vi "niDTS BT LE Rx Test  Initialize.vi"(0 "Dut Reference":T3, 5 "SystemTechnologyCatalog":refnum<class "niDTS SystemTechnologyCatalog.lvclass">, 7 "SystemDut":refnum<class "niDTS SystemDut.lvclass">, 9 "Logger Reference":T1, 11 "error in (no error)":errorcluster) -> (4 "RX Test Handle Out":T2, 6 "AllowAsync":bool=TRUE, 15 "error out":errorcluster)   [LabVIEW 2014, in "niDTS BT.lvlib"]
uses:
  niDTS BT.lvlib
  Framework/Dut/Includes/niDTS Dut INC Handle.ctl
  Framework/Dut/Objects/BASE_class/niDTS Dut.lvclass
  BDR Tx Test/Includes/niDTS BT Rx Test INC Handle.ctl
  Rx Test/Objects/BASE_class/niDTS BT Rx Test.lvclass
  TestStand/Station/Objects/SystemTechnologyCatalog/niDTS SystemTechnologyCatalog.lvclass
  TestStand/Station/Objects/SystemDut/niDTS SystemDut.lvclass
  Framework/Logger/Includes/niDTS Logger INC Handle.ctl
  Framework/Logger/Objects/BASE_class/niDTS Logger.lvclass
  Includes/niDTS BT INC Standard.ctl
  TestStand/niDTS TestStand.lvlib
  Framework/niDTS Framework.lvlib
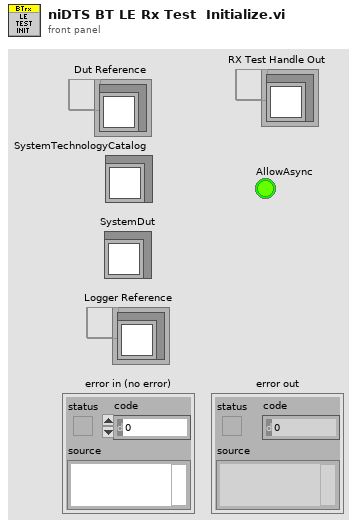
[diagram p1: front panel]
types:
  T1 = typedef "niDTS Framework.lvlib/niDTS Logger INC Handle.ctl" = refnum<data-value>
  T2 = typedef "niDTS BT.lvlib/niDTS BT Rx Test INC Handle.ctl" = refnum<data-value>
  T3 = typedef "niDTS Framework.lvlib/niDTS Dut INC Handle.ctl" = refnum<data-value>
  T4 = typedef "niDTS BT.lvlib/niDTS BT INC Standard.ctl" = enum16{"BDR", "EDR", "LE-TP"}
  T5 = typedef "niDTS TestStand.lvlib/niDTS TestStep INC Handle.ctl" = refnum<data-value>
  T6 = typedef "niDTS BT.lvlib/niDTS BT Rx Test INC Parameters.ctl" = cluster{"Channel":i32, "Dut Tx Power":dbl, "External Attenuation (dB)":dbl[], "Data Rate":enum16{"1", "2", "3"}, "Packet type":T7, "Payload Data":T8, "Carrier Mode":T9, "Number of Packets":i32, "Report Period (ms)":dbl, "BD ADDRESS":i64, "Dirty Tx":bool, "Corrupt Alternate CRC":bool, "Packet Header":T10, "Payload Header":T11, "Trigger":T12}
  T7 = typedef "niDTS BT.lvlib/niDTS BT INC Packet Type.ctl" = enum16{"NULL", "POLL", "FHS", "DM1", "DH1", "HV1", "HV2", "HV3", "EV3", "DV", "AUX1", "DM3", "DH3", "EV4", "EV5", "DM5", "DH5", "LE-TP"}
  T8 = typedef "niDTS BT.lvlib/niDTS BT Tx Test INC BD Payload Data.ctl" = enum16{"0", "1", "01", "00001111", "PN9", "AUTO"}
  T9 = typedef "niDTS BT.lvlib/niDTS BT Rx Test INC Carrier Mode.ctl" = enum16{"Burst", "Continuous"}
  T10 = typedef "niDTS BT.lvlib/niDTS BT Rx Test INC Packet Header.ctl" = cluster{"LT Address":i8, "Flow":i8, "ARQN":enum16{"NAK", "ACK"}, "Sequence Bit":i8}
  T11 = typedef "niDTS BT.lvlib/niDTS BT Rx Test INC Payload Header.ctl" = cluster{"LCh":i32, "HeaderFlowControlBit":bool, "Length (-1 AutoSet Max)":i32}
  T12 = typedef "niDTS BT.lvlib/niDTS BT DUT INC SG Trigger.ctl" = cluster{"TriggerEdge":enum16{"RISing", "FALLing"}, "TriggerSource":enum16{"IMMediate", "PFI 0", "PFI 1", "RTSI 0", "RTSI 1", "RTSI 2", "RTSI 3", "RTSI 4", "RTSI 5", "RTSI 6", "RTSI 7", "PXI STAR", "Software"}, "TriggerDelay (sec)":dbl, "TriggerTimeout (sec)":dbl}
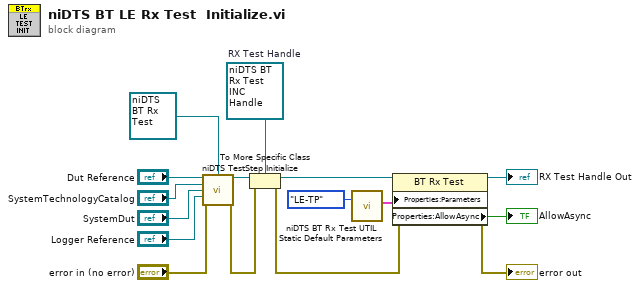
[diagram p0: block diagram]
diagram:
  w9 = T2 refnum  # RX Test Handle
  n1 = call "niDTS TestStep Initialize.vi"("Dut Handle"="Dut Reference", "Test Type"=refnum<class "niDTS BT Rx Test.lvclass"> refnum ("niDTS BT.lvlib:BT Rx Test"), "SystemTechnologyCatalog"="SystemTechnologyCatalog", "SystemDut"="SystemDut", "Logger Reference"="Logger Reference", "error in (no error)"="error in (no error)") -> ("Test Handle out"=w14:T5, "error out"=w13:errorcluster)  [unwired: 8 in]
  n2 = To More Specific Class(target class=w9, reference=w14, error in=w13) -> (specific class reference=w12:T2, error out=w11:errorcluster)
  n3 = call "niDTS BT Rx Test UTIL Static Default Parameters.vi"("BT Standard"=niDTS_BT_INC_Standard."LE-TP") -> ("Static Default Parameters"=w7:T6)  [unwired: 10 in]
  n4 = property class="BT Rx Test"(reference=w12, error in=w11, "Properties:Parameters"=w7) -> (reference out=→"RX Test Handle Out":T2, error out=→"error out":errorcluster, "Properties:AllowAsync"=→"AllowAsync":bool)
